vi "Session creator.vi"(8 "error in (no error)":errorcluster, 9 "Software version":dbl, 11 "Persistent In":T1) -> (0 "error out":errorcluster, 1 "Canceled":bool, 2 "Session properties":T2, 3 "Created file":path, 5 "Persistent Out":T1)   [LabVIEW 2019]
doc: "Handles creation of a new session, displays a GUI window"
uses:
  Type defs/Session properties Type Def.ctl
  Type defs/Persistent Type Def.ctl
  <vilib>/Utility/miscctls.llb/LVPointTypeDef.ctl
  <vilib>/Utility/sysdir.llb/System Directory Type.ctl
panel:
  in  "User":string(combo) caption="Combo Box"
  in  "Cancel":bool
  in  "Apply":bool
  in  "Path":path
  in  "Comment":string
  in  "Session name":string
  in  "Internal structure":enum32{"Binary", "Text based"}(radio)
  # "Measurement session creator"
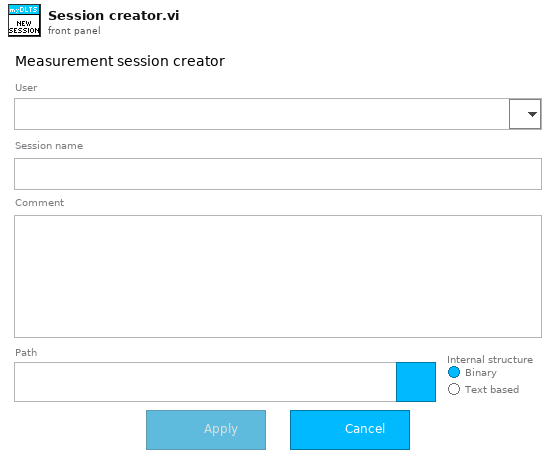
[diagram p1: front panel]
types:
  T1 = typedef "Persistent Type Def.ctl" = cluster{"Last file":path, "Last user":string, "Users":cluster{"User":string, "Authors directory":path}[]}
  T2 = typedef "Session properties Type Def.ctl" = cluster{"Session name":string, "Comment":string, "User":string, "Software version":dbl, "Created":timestamp, "Modified":timestamp, "Binary":bool, "GUID":string}
  T3 = enum8{"Enabled", "Disabled", "Disabled and Grayed Out"}
  T4 = typedef "LVPointTypeDef.ctl" = cluster{"Horizontal":i16, "Vertical":i16}
  T5 = cluster{"User":string, "Authors directory":path}[]
  T6 = typedef "System Directory Type.ctl" = i32
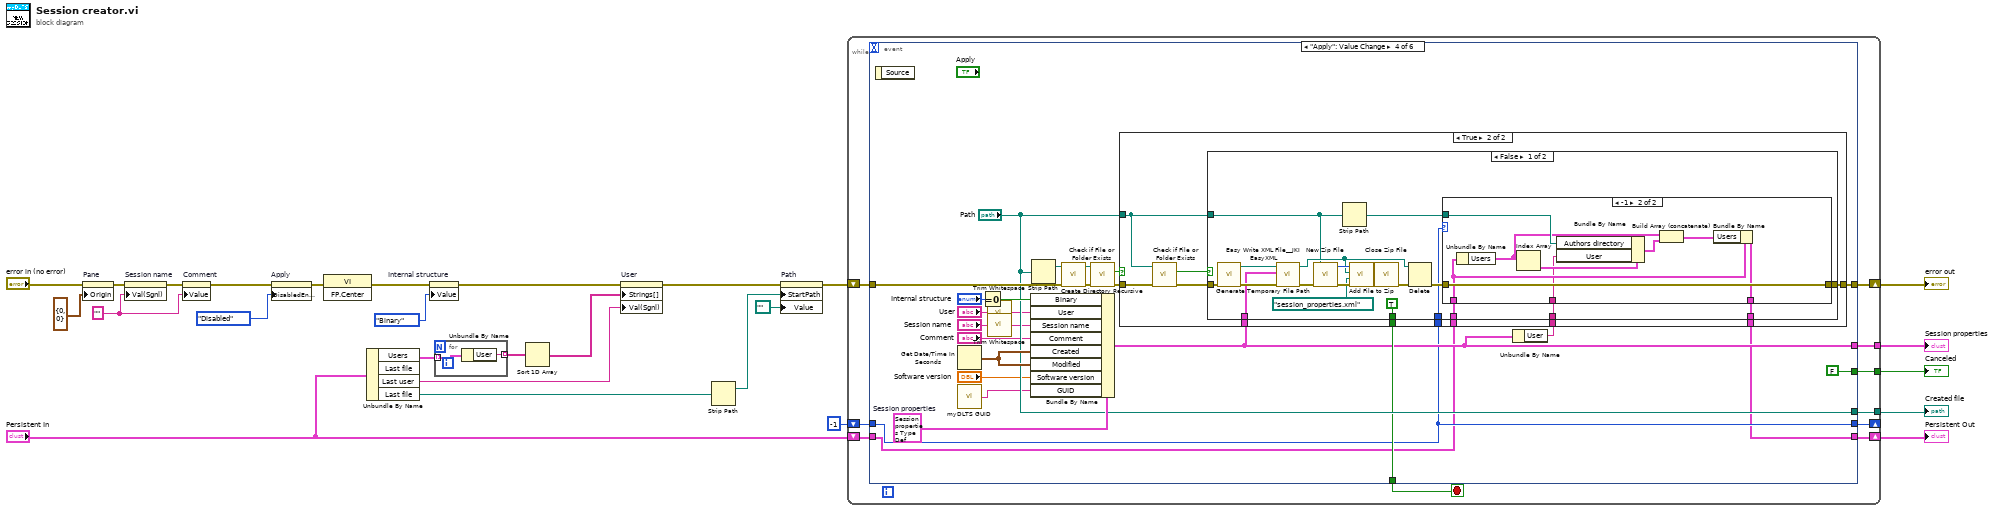
[diagram p0: block diagram]
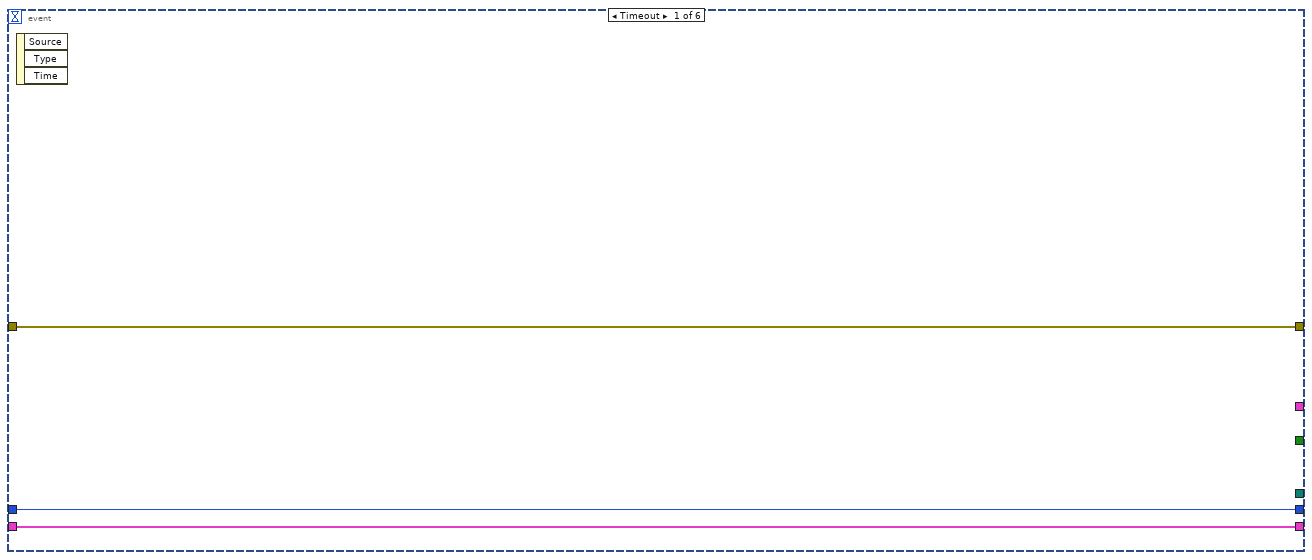
[diagram p2: hidden frame]
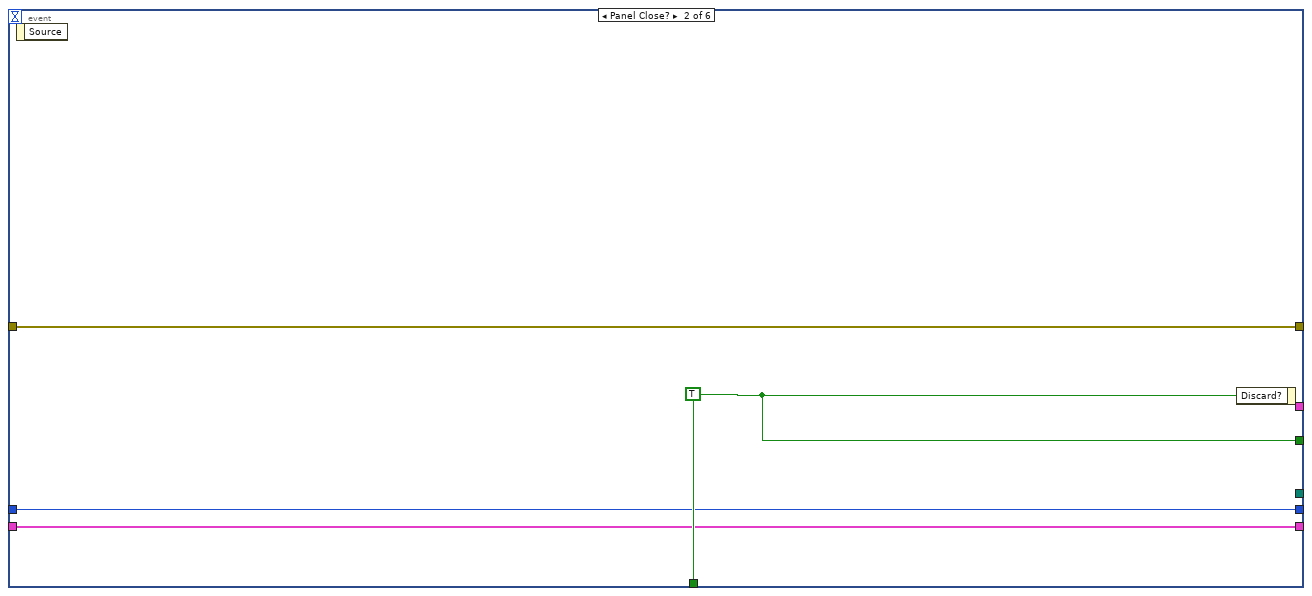
[diagram p3: hidden frame]
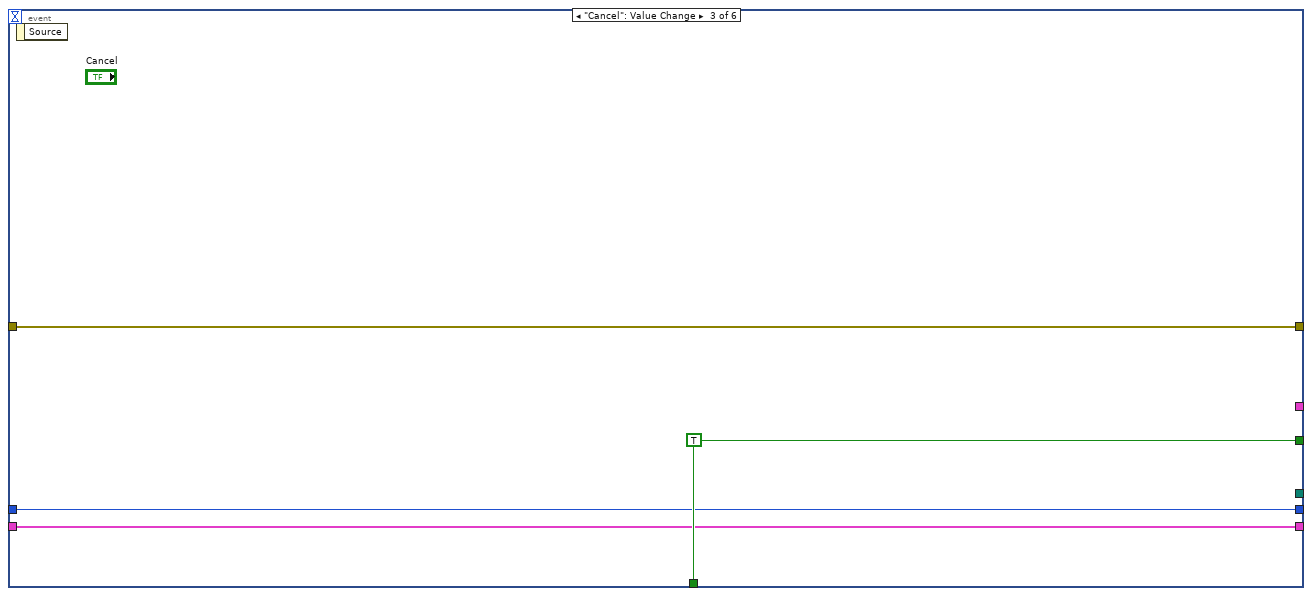
[diagram p4: hidden frame]
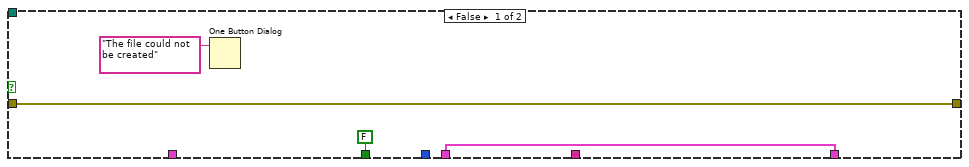
[diagram p5: hidden frame]
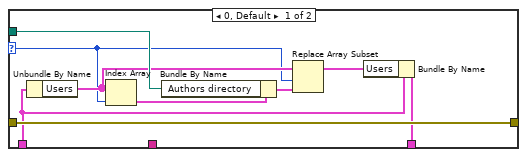
[diagram p6: hidden frame]
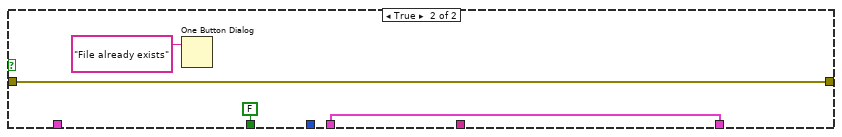
[diagram p7: hidden frame]
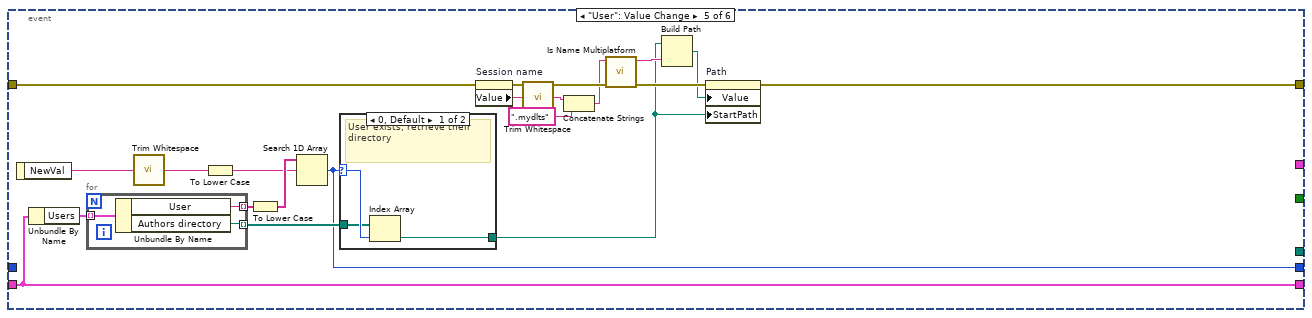
[diagram p8: hidden frame]
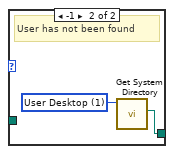
[diagram p9: hidden frame]
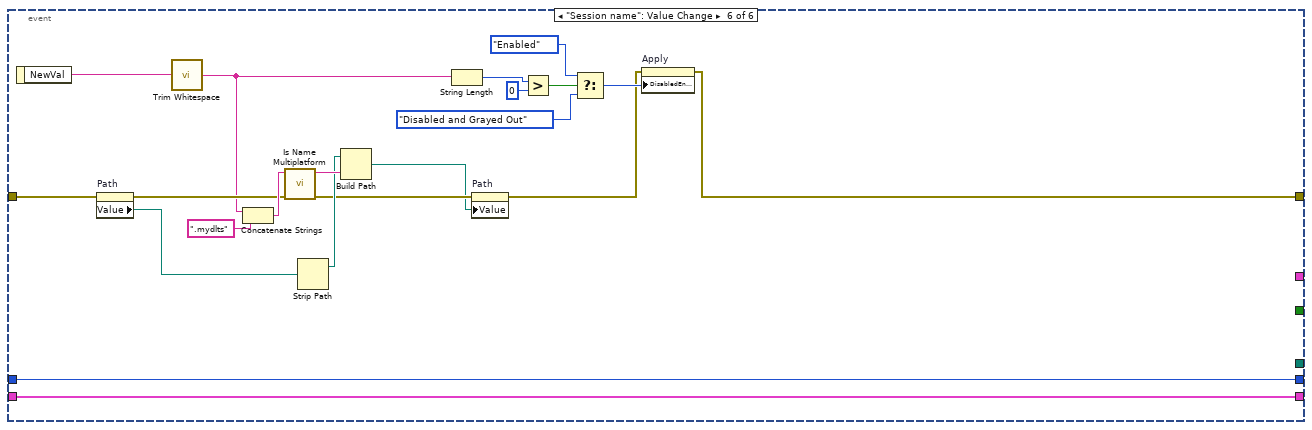
[diagram p10: hidden frame]
diagram:
  w16 = "" ("Value (Signaling)")
  n1 = property on="Pane" class="Pane"(error in="error in (no error)", "Origin"=T4 {"Horizontal"=0, "Vertical"=0}) -> (error out=w26:errorcluster)  [unwired: 1 in, 1 out]
  n2 = property on="Session name" class="Str"(error in=w26, "Val(Sgnl)"=w16) -> (error out=w19:errorcluster)  [unwired: 1 in, 1 out]
  n3 = property on="Comment" class="Str"(error in=w19, "Value"=w16) -> (error out=w17:errorcluster)  [unwired: 1 in, 1 out]
  n4 = property on="Apply" class="Bool"(error in=w17, "DisabledEnum"=T3."Disabled" ("Disabled")) -> (error out=w14:errorcluster)  [unwired: 1 in, 1 out]
  n5 = invoke class="VI" method="FP.Center"(error in=w14) -> (error out=w13:errorcluster)  [unwired: 2 in, 2 out]
  n6 = Unbundle By Name("Persistent In") -> ("Users"=w10:T5, "Last user"=w7:string, "Last file"=w6:path)  [unwired: 1 out]
  n7 = property on="Internal structure" class="RadioBtnsControl (strict)"(error in=w13, "Value"=enum32{"Binary", "Text based"}."Binary" ("Internal structure")) -> (error out=w5:errorcluster)  [unwired: 1 in, 1 out]
  n8 = for {
    tunnel: w10 -> [w29] mode=indexing
    tunnel: [w28] -> w9 mode=indexing
    n9 = Unbundle By Name(w29) -> ("User"=w28:string)
  }
  n10 = Sort 1D Array(array=w9) -> (sorted array=w8:string[])
  n11 = property on="User" class="CmbBox"(error in=w5, "Strings[]"=w8, "Val(Sgnl)"=w7) -> (error out=w4:errorcluster)  [unwired: 1 in, 1 out]
  n12 = Strip Path(path=w6) -> (stripped path=w11:path)  [unwired: 1 out]
  n13 = property on="Path" class="Path"(error in=w4, "StartPath"=w11, "Value"=path "" ("File Path")) -> (error out=w22:errorcluster)  [unwired: 1 in, 1 out]
  n14 = while {
    tunnel: [w38] -> w27
    shift-right: [w36] -> w24
    shift-left: w22 -> [w37]
    tunnel: [w35] -> w21
    tunnel: [w34] -> w20
    shift-right: [w32] -> w3
    shift-left: "Persistent In" -> [w33]
    shift-right: [w31] -> _
    shift-left: -1 ("index of element") -> [w30]
    stop <- w39 stop-if-true
    n15 = event shown="[3] \"Apply\": Value Change" {
      selector: _ -> [_ _ _ _ _ _]
      dyn-events: _ -> [_ _ _ _ _ _]
      timeout: _ -> [_ _ _ _ _ _]
      tunnel: [_ w46 w50 w60 _ _] -> w39
      tunnel: [_ w46 w50 FALSE ("Discard?") _ _] -> w38
      tunnel: w37 -> [w42 w45 w49 w74 w137 w172]
      tunnel: [w42 w45 w49 w67 w147 w179] -> w36
      tunnel: [_ _ _ w56 _ _] -> w35
      tunnel: [_ _ _ "Path" _ _] -> w34
      tunnel: w33 -> [w40 w43 w47 w53 w149 w163]
      tunnel: [w40 w43 w47 w52 w149 w163] -> w32
      tunnel: [w41 w44 w48 w54 w148 w164] -> w31
      tunnel: w30 -> [w41 w44 w48 w54 _ w164]
      event Timeout {
        n16 = event-data() -> ()  [unwired: 1 in, 3 out]
      }
      event Panel Close? {
        w46 = TRUE ("Discard?")
        n17 = event-data() -> ()  [unwired: 1 in, 1 out]
        n18 = event-data("Discard?"=w46) -> ()  [unwired: 1 in, 1 out]
      }
      event "Cancel": Value Change {
        w50 = TRUE ("Discard?")
        n19 = event-data() -> ()  [unwired: 1 in, 1 out]
      }
      event "Apply": Value Change {
        w69 = T2 {"Session name"="", "Comment"="", "User"="", "Software version"=0.0, "Created"=timestamp(0 s since 1904-01-01), "Modified"=timestamp(0 s since 1904-01-01), "Binary"=FALSE, "GUID"=""}  # Session properties
        n20 = event-data() -> ()  [unwired: 1 in, 1 out]
        n21 = Get Date/Time In Seconds() -> (seconds since 1Jan1904=w68:timestamp)
        n22 = call "myDLTS GUID.vi"() -> ("GUID"=w51:string)  [unwired: 1 in]
        n23 = Equal To 0?(x="Internal structure") -> (x = 0?=w65:bool)
        n24 = call <vilib>:"Trim Whitespace.vi"("string"="User") -> ("trimmed string"=w57:string)  [unwired: 1 in]
        n25 = call <vilib>:"Trim Whitespace.vi"("string"="Session name") -> ("trimmed string"=w61:string)  [unwired: 1 in]
        n26 = Bundle By Name(cluster=w69, "Binary"=w65, "User"=w57, "Session name"=w61, "Comment"="Comment", "Created"=w68, "Modified"=w68, "Software version"="Software version", "GUID"=w51) -> (w56:T2)
        n27 = Strip Path(path="Path") -> (stripped path=w75:path)  [unwired: 1 out]
        n28 = call <vilib>:"Create Directory Recursive.vi"("error in (no error)"=w74, "directory"=w75) -> ("error out"=w73:errorcluster, "directory copy"=w72:path)  [unwired: 3 in, 1 out]
        n29 = call <vilib>:"Check if File or Folder Exists.vi"("error in (no error)"=w73, "path"=w72) -> ("error out"=w71:errorcluster, "file or folder exists?"=w70:bool)  [unwired: 7 in, 1 out]
        n30 = Unbundle By Name(w56) -> ("User"=w55:string)
        n31 = case shown="True" w70 {
          tunnel: "Path" -> [_ w88]
          tunnel: w71 -> [w80 w90]
          tunnel: [w80 w91] -> w67
          tunnel: w56 -> [_ w87]
          tunnel: [FALSE ("Discard?") w85] -> w60
          tunnel: w55 -> [_ w84]
          tunnel: w54 -> [_ w83]
          tunnel: w53 -> [w77 w82]
          tunnel: [w77 w81] -> w52
          frame False {
            n32 = One Button Dialog(message="The file could not be created") -> ()  [unwired: 1 in, 1 out]
          }
          frame True {
            n33 = call <vilib>:"Check if File or Folder Exists.vi"("error in (no error)"=w90, "path"=w88) -> ("error out"=w89:errorcluster, "file or folder exists?"=w86:bool)  [unwired: 7 in, 1 out]
            n34 = case shown="False" w86 {
              tunnel: w88 -> [w95 _]
              tunnel: w89 -> [w108 w134]
              tunnel: [w96 w134] -> w91
              tunnel: w87 -> [w101 _]
              tunnel: [TRUE ("Discard?") FALSE ("Discard?")] -> w85
              tunnel: w84 -> [w93 _]
              tunnel: w83 -> [w98 _]
              tunnel: w82 -> [w97 w131]
              tunnel: [w94 w131] -> w81
              frame False {
                n35 = call <vilib>:"Generate Temporary File Path.vi"("error in (no error)"=w108) -> ("error out"=w105:errorcluster, "Unique Temporary File Path"=w102:path)  [unwired: 9 in]
                n36 = call <vilib>:"Easy Write XML File__JKI EasyXML.vi"("error in (no error)"=w105, "LabVIEW Data"=w101, "XML File Path"=w102) -> ("error out"=w104:errorcluster, "XML File Path (duplicate)"=w103:path)  [unwired: 7 in]
                n37 = call <vilib>:"New Zip File.vi"("error in (no error)"=w104, "target"=w95) -> ("error out"=w109:errorcluster, "zip file out"=w112:i64)  [unwired: 3 in, 1 out]
                n38 = Strip Path(path=w95) -> (stripped path=w92:path)  [unwired: 1 out]
                n39 = call <vilib>:"Add File to Zip.vi"("error in (no error)"=w109, "destination path in zip"=path "session_properties.xml", "source file path"=w103, "zip file in"=w112) -> ("error out"=w110:errorcluster, "zip file out"=w111:i64)  [unwired: 6 in]
                n40 = call <vilib>:"Close Zip File.vi"("error in (no error)"=w110, "zip file in"=w111) -> ("error out"=w106:errorcluster)  [unwired: 5 in]
                n41 = Delete(path (use dialog)=w103, error in=w106) -> (error out=w99:errorcluster)  [unwired: 3 in, 2 out]
                n42 = case shown="-1" w98 {
                  selector: w98 -> [w117 _]
                  tunnel: w99 -> [w121 w130]
                  tunnel: w97 -> [w115 w125]
                  tunnel: [w121 w130] -> w96
                  tunnel: w92 -> [w119 w128]
                  tunnel: [w113 w123] -> w94
                  tunnel: w93 -> [_ w122]
                  frame 0, Default {
                    n43 = Unbundle By Name(w115) -> ("Users"=w118:T5)
                    n44 = Index Array(array=w118, index=w117) -> (element=w120:cluster{"User":string, "Authors directory":path})
                    n45 = Bundle By Name(cluster=w120, "Authors directory"=w119) -> (w116:cluster{"User":string, "Authors directory":path})
                    n46 = Replace Array Subset(array=w118, new element=w116, index=w117) -> (w114:T5)
                    n47 = Bundle By Name(cluster=w115, "Users"=w114) -> (w113:T1)
                  }
                  frame -1 {
                    n48 = Unbundle By Name(w125) -> ("Users"=w127:T5)
                    n49 = Index Array(array=w127) -> (element=w129:cluster{"User":string, "Authors directory":path})  [unwired: 1 in]
                    n50 = Bundle By Name(cluster=w129, "Authors directory"=w128, "User"=w122) -> (w126:cluster{"User":string, "Authors directory":path})
                    n51 = Build Array (concatenate)(w127, w126) -> (w124:T5)
                    n52 = Bundle By Name(cluster=w125, "Users"=w124) -> (w123:T1)
                  }
                }
              }
              frame True {
                n53 = One Button Dialog(message="File already exists") -> ()  [unwired: 1 in, 1 out]
              }
            }
          }
        }
      }
      event "User": Value Change {
        n54 = event-data() -> ("NewVal"=w136:string)  [unwired: 1 in]
        n55 = Unbundle By Name(w149) -> ("Users"=w154:T5)
        n56 = for {
          tunnel: w154 -> [w162] mode=indexing
          tunnel: [w161] -> w153 mode=indexing
          tunnel: [w160] -> w150 mode=indexing
          n57 = Unbundle By Name(w162) -> ("User"=w161:string, "Authors directory"=w160:path)
        }
        n58 = call <vilib>:"Trim Whitespace.vi"("string"=w136) -> ("trimmed string"=w135:string)  [unwired: 1 in]
        n59 = To Lower Case(string=w135) -> (all lower case string=w151:string)
        n60 = To Lower Case(string=w153) -> (all lower case string=w152:string[])
        n61 = Search 1D Array(1D array=w152, element=w151) -> (index of element=w148:i32)  [unwired: 1 in]
        n62 = case shown="0, Default" w148 {
          selector: w148 -> [w157 _]
          tunnel: w150 -> [w156 _]
          tunnel: [w155 w158] -> w138
          frame 0, Default {
            # "User exists, retrieve their directory"
            n63 = Index Array(array=w156, index=w157) -> (element=w155:path)
          }
          frame -1 {
            w159 = T6 1 items=["User Home"=0, "User Desktop"=1, "User Documents"=2, "User Application Data"=3, "User Preferences"=4, "User Temporary"=5, "Public Documents"=6, "Public Application Data"=7, "Public Preferences"=8, "Public Cache"=13, "System Core Libraries"=9, "System Installed Libraries"=10, "Application Files"=11, "Boot Volume Root"=12] ("system directory type")
            # "User has not been found"
            n64 = call <vilib>:"Get System Directory.vi"("system directory type"=w159) -> ("system directory"=w158:path)  [unwired: 10 in]
          }
        }
        n65 = property on="Session name" class="Str"(error in=w137) -> (error out=w146:errorcluster, "Value"=w142:string)  [unwired: 1 in, 1 out]
        n66 = call <vilib>:"Trim Whitespace.vi"("string"=w142) -> ("trimmed string"=w143:string)  [unwired: 1 in]
        n67 = Concatenate Strings(w143, ".mydlts" ("string")) -> (w145:string)
        n68 = call <vilib>:"Is Name Multiplatform.vi"("error in (no error)"=w146, "filename"=w145) -> ("error out"=w140:errorcluster, "suggested filename"=w144:string)  [unwired: 5 in, 3 out]
        n69 = Build Path(base path=w138, name or relative path=w144) -> (appended path=w139:path)
        n70 = property on="Path" class="Path"(error in=w140, "Value"=w139, "StartPath"=w138) -> (error out=w147:errorcluster)  [unwired: 1 in, 1 out]
      }
      event "Session name": Value Change {
        n71 = event-data() -> ("NewVal"=w181:string)  [unwired: 1 in]
        n72 = property on="Path" class="Path"(error in=w172) -> (error out=w170:errorcluster, "Value"=w175:path)  [unwired: 1 in, 1 out]
        n73 = call <vilib>:"Trim Whitespace.vi"("string"=w181) -> ("trimmed string"=w169:string)  [unwired: 1 in]
        n74 = Concatenate Strings(w169, ".mydlts" ("string")) -> (w171:string)
        n75 = call <vilib>:"Is Name Multiplatform.vi"("error in (no error)"=w170, "filename"=w171) -> ("error out"=w167:errorcluster, "suggested filename"=w174:string)  [unwired: 5 in, 3 out]
        n76 = Strip Path(path=w175) -> (stripped path=w168:path)  [unwired: 1 out]
        n77 = Build Path(base path=w168, name or relative path=w174) -> (appended path=w165:path)
        n78 = String Length(string=w169) -> (length=w177:i32)
        n79 = property on="Path" class="Path"(error in=w167, "Value"=w165) -> (error out=w166:errorcluster)  [unwired: 1 in, 1 out]
        n80 = Greater?(x=w177, y=0) -> (0:w176:bool)
        n81 = Select(t=T3."Enabled" ("Disabled"), s=w176, f=T3."Disabled and Grayed Out") -> (s? t:f=w180:T3)
        n82 = property on="Apply" class="Bool"(error in=w166, "DisabledEnum"=w180) -> (error out=w179:errorcluster)  [unwired: 1 in, 1 out]
      }
    }
  }
  "Canceled" <- w27
  "error out" <- w24
  "Session properties" <- w21
  "Created file" <- w20
  "Persistent Out" <- w3
